vi "piezoUSBWriteTest.vi"() -> ()   [LabVIEW 2017]
panel:
  in  "stop":bool
  in  "position":dbl
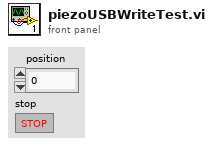
[diagram p1: front panel]
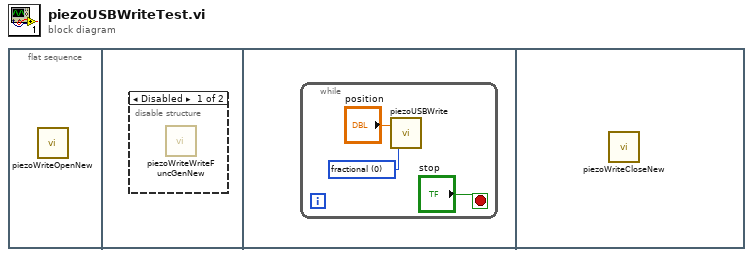
[diagram p0: block diagram]
diagram:
  n1 = flat-sequence {
    frame #0 {
      n2 = call "piezoWriteOpenNew.vi"() -> ()  [unwired: 2 in]
    }
    frame #1 {
      n3 = disable-structure shown="Disabled" {
        frame Disabled {
          n4 = call "piezoWriteWriteFuncGenNew.vi"() -> ()  [unwired: 12 in]
        }
        frame Enabled {
        }
      }
    }
    frame #2 {
      n5 = while {
        stop <- "stop" stop-if-true
        w2 = u16 0 items=["fractional", "voltage (V)", "position (um)"] ("mode")
        n6 = call "piezoUSBWrite.vi"("mode"=w2, "position"="position") -> ()  [unwired: 1 in]
      }
    }
    frame #3 {
      n7 = call "piezoWriteCloseNew.vi"() -> ()  [unwired: 1 in]
    }
  }
